vi "ConvertMFCDisplayStateToCSVString.vi"(11 "MFC Valve State":T1) -> (3 "CSV String":string)   [LabVIEW 2012]
uses:
  MFCDisplayValveState.ctl
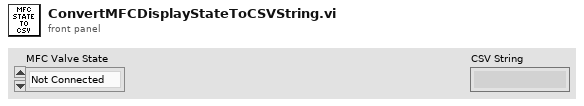
[diagram p1: front panel]
types:
  T1 = typedef "MFCDisplayValveState.ctl" = enum16{"Not Connected", "Automatic", "Closed", "Purge"}
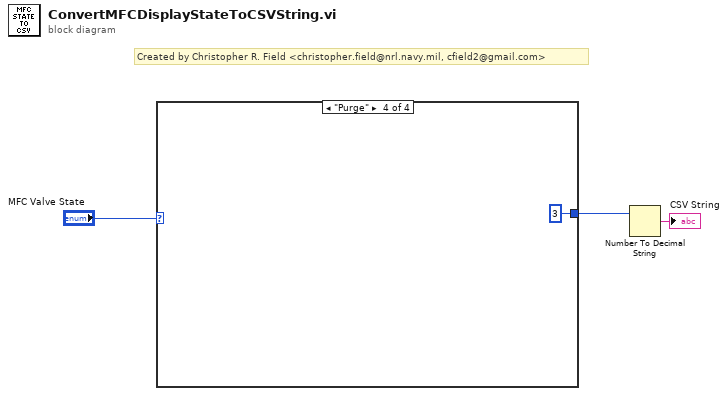
[diagram p0: block diagram]
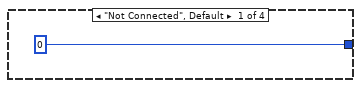
[diagram p2: hidden frame]
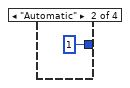
[diagram p3: hidden frame]
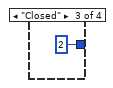
[diagram p4: hidden frame]
diagram:
  # "Created by Christopher R. Field <christopher.field@nrl.navy.mil, cfield2@gmail.com>"
  n1 = case shown="\"Purge\"" "MFC Valve State" {
    tunnel: [0 1 2 3] -> w2
    frame "Not Connected", Default {
    }
    frame "Automatic" {
    }
    frame "Closed" {
    }
    frame "Purge" {
    }
  }
  n2 = Number To Decimal String(number=w2) -> (decimal integer string=→"CSV String":string)  [unwired: 1 in]
